vi "AdjustLauncherRPM.vi"(9 "Current RPM":dbl) -> (1 "New RPM":dbl)   [LabVIEW 2012]
uses:
  Robot Global Data.vi
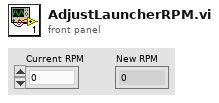
[diagram p1: front panel]
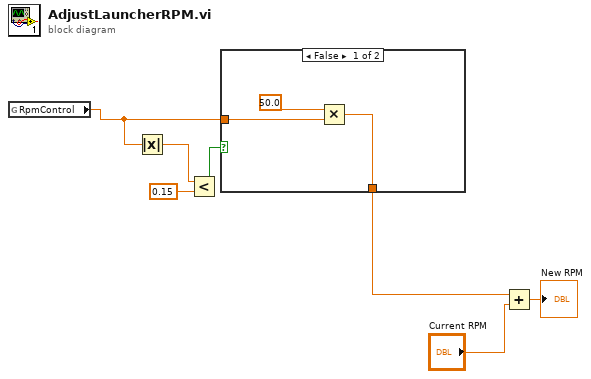
[diagram p0: block diagram]
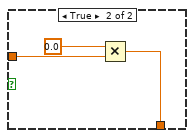
[diagram p2: hidden frame]
diagram:
  n1 = global read "Robot Global Data.vi" "RpmControl"() -> (w1:dbl)
  n2 = Absolute Value(x=w1) -> (abs(x)=w4:dbl)
  n3 = Less?(x=w4, y=0.15) -> (x < y?=w2:bool)
  n4 = case shown="False" w2 {
    tunnel: [w10 w13] -> w5
    tunnel: w1 -> [w8 w12]
    frame False {
      n5 = Multiply(x=50.0, y=w8) -> (x*y=w10:dbl)
    }
    frame True {
      n6 = Multiply(x=0.0, y=w12) -> (x*y=w13:dbl)
    }
  }
  n7 = Add(x=w5, y="Current RPM") -> (x+y=→"New RPM":dbl)
